vi "chart axis set name range lv.vi"(7 "col":u16, 8 "error in (no error)":errorcluster, 9 "row":u32, 10 "sheetname":string, 11 "axis":u32) -> (0 "error out":errorcluster)   [LabVIEW 2015, in "xlsxwriter.lvlib"]
doc: "void chart_axis_set_name_range_lv(lxw_chart_axis axis, const char *sheetname, lxw_row_t row, lxw_col_t col);"
uses:
  xlsxwriter.lvlib
  xlsxwriter.dll
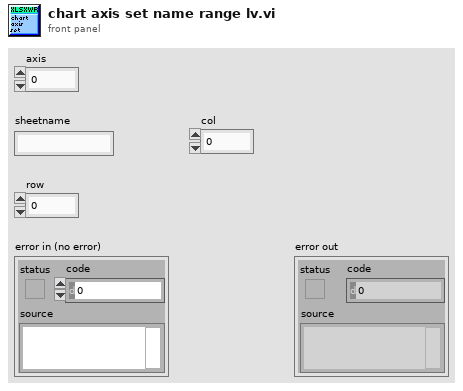
[diagram p1: front panel]
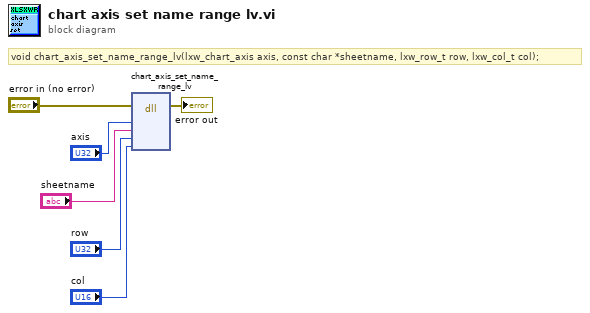
[diagram p0: block diagram]
diagram:
  # "void chart_axis_set_name_range_lv(lxw_chart_axis axis, const char *sheetname, lxw_row_t row, lxw_col_t col);"
  n1 = dll-call lib="C:/Users/WDAGUtilityAccount/Desktop/lv_vis_added_cell/xlsxwriter.*" fn="chart_axis_set_name_range_lv"(error in="error in (no error)", "axis"="axis", "sheetname"="sheetname", "row"="row", "col"="col") -> (error out=→"error out":errorcluster)  [unwired: 7 in, 1 out]
